vi "ODX_Rechenbefehl.vi"(9 "Operand in":u32, 11 "operation":T1 {"Wert" format="%.0x"}) -> (1 "Operand out":u32, 2 "Carry":bool)   [LabVIEW 2012]
uses:
  Typedefs/Diagnose_SA2_Operation_ENUM.ctl
  Typedefs/Diagnose_SA2_Rechnenbefehl.ctl
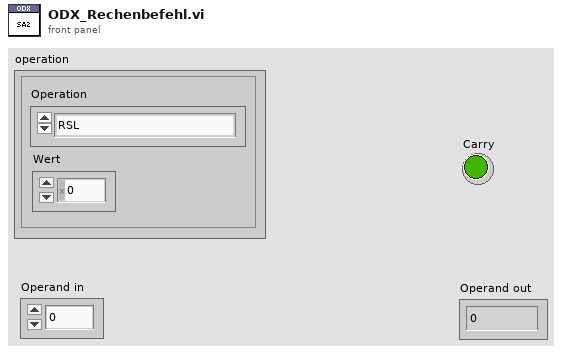
[diagram p1: front panel]
types:
  T1 = typedef "Diagnose_SA2_Rechnenbefehl.ctl" = cluster{"Operation":T2, "Wert":u32}
  T2 = typedef "Diagnose_SA2_Operation_ENUM.ctl" = enum16{"RSL", "RSR", "ADD", "SUB", "EOR", "Durchläufe", "NEXT", "BCC", "BRA", "Fertig"}
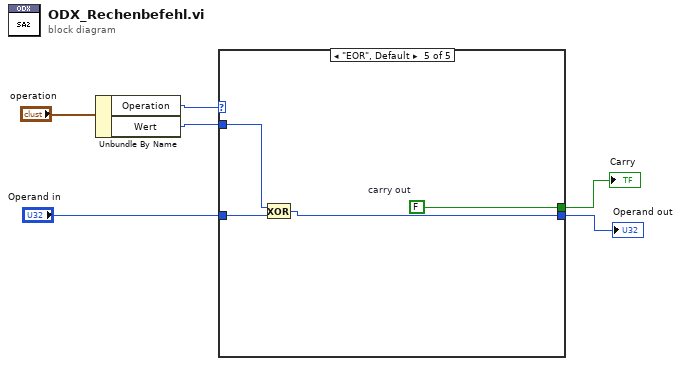
[diagram p0: block diagram]
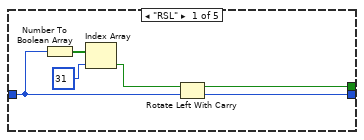
[diagram p2: hidden frame]
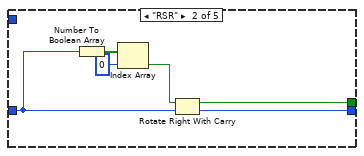
[diagram p3: hidden frame]
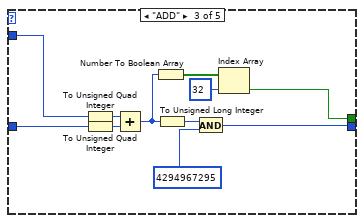
[diagram p4: hidden frame]
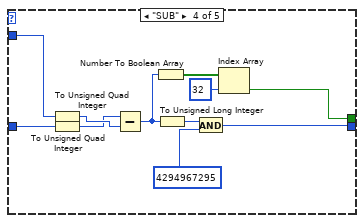
[diagram p5: hidden frame]
diagram:
  n1 = Unbundle By Name("operation") -> ("Operation"=w4:T2, "Wert"=w5:u32)
  n2 = case shown="\"EOR\", Default" w4 {
    tunnel: w5 -> [_ _ w29 w40 w44]
    tunnel: "Operand in" -> [w7 w13 w28 w39 w43]
    tunnel: [w9 w16 w26 w37 w42] -> w1
    tunnel: [w8 w15 w22 w33 w41] -> w2
    frame "RSL" {
      n3 = Number To Boolean Array(number=w7) -> (Boolean array=w12:bool[])
      n4 = Index Array(array=w12, index=31) -> (element=w10:bool)
      n5 = Rotate Left With Carry(2:w7, 3:w10) -> (0:w9:u32, 1:w8:bool)
    }
    frame "RSR" {
      n6 = Number To Boolean Array(number=w13) -> (Boolean array=w18:bool[])
      n7 = Index Array(array=w18, index=0) -> (element=w14:bool)
      n8 = Rotate Right With Carry(2:w13, 3:w14) -> (0:w16:u32, 1:w15:bool)
    }
    frame "ADD" {
      n9 = To Unsigned Quad Integer(1:w29) -> (0:w21:u64)
      n10 = To Unsigned Quad Integer(1:w28) -> (0:w20:u64)
      n11 = Add(x=w21, y=w20) -> (x+y=w25:u64)
      n12 = Number To Boolean Array(number=w25) -> (Boolean array=w24:bool[])
      n13 = To Unsigned Long Integer(number=w25) -> (unsigned 32bit integer=w19:u32)
      n14 = And(x=w19, y=u32 4294967295) -> (x .and. y?=w26:u32)
      n15 = Index Array(array=w24, index=32) -> (element=w22:bool)
    }
    frame "SUB" {
      n16 = To Unsigned Quad Integer(1:w40) -> (0:w32:u64)
      n17 = To Unsigned Quad Integer(1:w39) -> (0:w31:u64)
      n18 = Subtract(x=w31, y=w32) -> (x-y=w36:u64)
      n19 = Number To Boolean Array(number=w36) -> (Boolean array=w35:bool[])
      n20 = To Unsigned Long Integer(number=w36) -> (unsigned 32bit integer=w30:u32)
      n21 = And(x=w30, y=u32 4294967295) -> (x .and. y?=w37:u32)
      n22 = Index Array(array=w35, index=32) -> (element=w33:bool)
    }
    frame "EOR", Default {
      w41 = FALSE  # carry out
      n23 = Exclusive Or(1:w43, 2:w44) -> (0:w42:u32)
    }
  }
  "Carry" <- w2
  "Operand out" <- w1
